vi "onDestroy.vi"(8 "error in (no error)":errorcluster, 11 "Camera.Simulated":refnum<class "Camera.Simulated.lvclass">) -> (0 "error out":errorcluster, 3 "Camera.Simulated out":refnum<class "Camera.Simulated.lvclass">)   [LabVIEW 2015, in "Camera.Simulated.lvclass"]
doc: "JKI State Machine Objects (SMO) 1.0.4.18\nJKI - JKI\nCopyright (c) 2016, JKI"
uses:
  Camera.Simulated.lvclass
  Camera/Camera.lvclass
  <vilib>/JKI/JKI SMO/SMO/SMO.lvclass
panel:
  # "For instructions on how to use the JKI State Machine Objects, examples and video tutorials, visit:\nhttp://jki.net/state-machine-objects/\n\nJKI State Machine Objects™\nhttp://jki.net/state-machine-objects/\nCopyright (C) 2005-2015, JKI <info@jki.net>\nALL RIGHTS RESERVED"
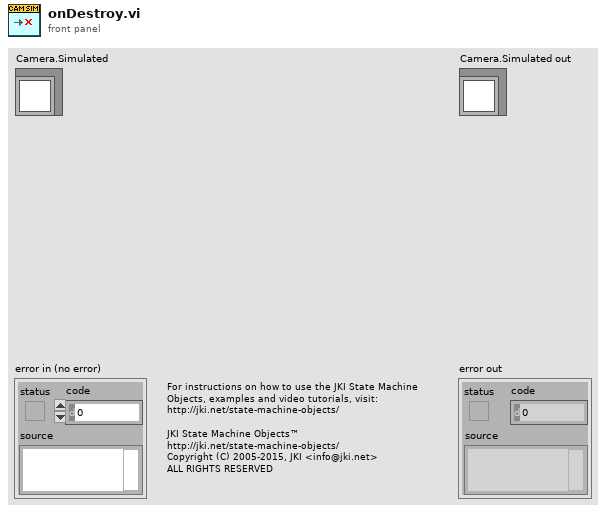
[diagram p1: front panel]
types:
  T1 = typedef "Camera.Simulated.lvclass/Dependencies--Cluster.ctl" = cluster{"CircularBuffer.ImageData":refnum<class "CircularBuffer.ImageData.lvclass">}
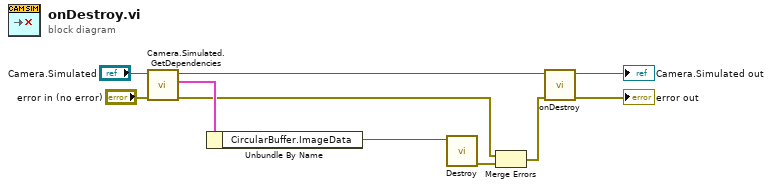
[diagram p0: block diagram]
diagram:
  n1 = call "Camera.Simulated.GetDependencies.vi"("error in (no error)"="error in (no error)", "Camera.Simulated"="Camera.Simulated") -> ("error out"=w6:errorcluster, "Dependencies"=w9:T1, "Camera.Simulated"=w10:refnum<class "Camera.Simulated.lvclass">)  [unwired: 7 in]
  n2 = Unbundle By Name(w9) -> ("CircularBuffer.ImageData"=w8:refnum<class "CircularBuffer.ImageData.lvclass">)
  n3 = call <vilib>:"Destroy.vi"("SMO"=w8) -> ("error out"=w7:errorcluster)  [unwired: 10 in]
  n4 = Merge Errors(w6, w7) -> (w5:errorcluster)
  n5 = call-parent "onDestroy.vi"("error in (no error)"=w5, "Camera"=w10) -> ("error out"=→"error out":errorcluster, "Camera out"=→"Camera.Simulated out":refnum<class "Camera.Simulated.lvclass">)  [unwired: 8 in]
